vi "Generate Data.vi"(8 "Error In":errorcluster, 11 "Data in":refnum<class "Data.lvclass">) -> (0 "Error Out":errorcluster, 3 "Data out":refnum<class "Data.lvclass">)   [LabVIEW 2020, in "Data.lvclass"]
doc: "The method is a over riding method that generates different data for different data types."
uses:
  Data.lvclass
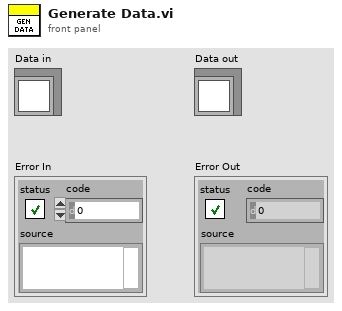
[diagram p1: front panel]
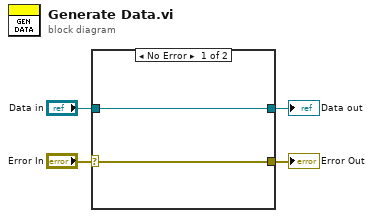
[diagram p0: block diagram]
diagram:
  n1 = case shown="No Error" "Error In" {
    selector: "Error In" -> [w5 w8]
    tunnel: [w5 w8] -> w3
    tunnel: [w6 w7] -> w1
    tunnel: "Data in" -> [w6 w7]
    frame No Error {
    }
    frame Error {
    }
  }
  "Error Out" <- w3
  "Data out" <- w1
